vi "DO Tristate with DI.vi"() -> ()   [LabVIEW 2011]
uses:
  <vilib>/DAQmx/write.llb/DAQmx Write (Digital Bool 1Line 1Point).vi
  <vilib>/DAQmx/read.llb/DAQmx Read (Digital Bool 1Line 1Point).vi
  <vilib>/DAQmx/create/channels.llb/DAQmx Create Channel (DO-Digital Output).vi
  <vilib>/DAQmx/miscellaneous.llb/DAQmx Fill In Error Info.vi
  <vilib>/DAQmx/create/channels.llb/DAQmx Create Channel (DI-Digital Input).vi
panel:
  in  "State to Write":enum16{"Tristate", "High", "Low"}(ring)
  out "data":bool
  in  "Digital Line":tag
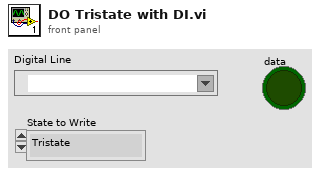
[diagram p1: front panel]
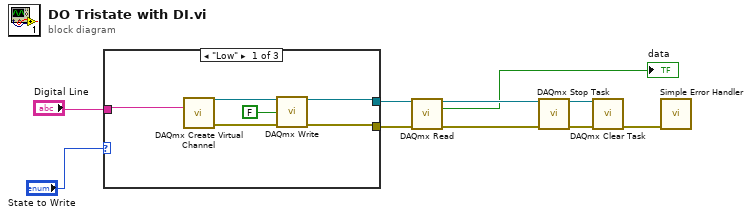
[diagram p0: block diagram]
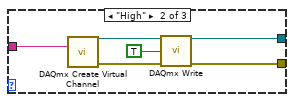
[diagram p2: hidden frame]
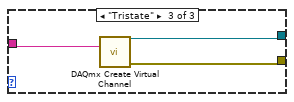
[diagram p3: hidden frame]
diagram:
  n1 = case shown="\"Low\"" "State to Write" {
    tunnel: [w12 w22 w24] -> w8
    tunnel: [w11 w21 w23] -> w7
    tunnel: "Digital Line" -> [w13 w19 w25]
    frame "Low" {
      n2 = call-poly <vilib>:"DAQmx Create Virtual Channel.vi"("lines"=w13) -> ("task out"=w14:refnum<k21>, "error out"=w15:errorcluster)  [unwired: 13 in]
      n3 = call-poly <vilib>:"DAQmx Write.vi"("task/channels in"=w14, "data"=FALSE, "error in"=w15) -> ("task out"=w12:refnum<k21>, "error out"=w11:errorcluster)  [unwired: 10 in, 1 out]
    }
    frame "High" {
      n4 = call-poly <vilib>:"DAQmx Create Virtual Channel.vi"("lines"=w19) -> ("task out"=w17:refnum<k21>, "error out"=w18:errorcluster)  [unwired: 13 in]
      n5 = call-poly <vilib>:"DAQmx Write.vi"("task/channels in"=w17, "data"=TRUE, "error in"=w18) -> ("task out"=w22:refnum<k21>, "error out"=w21:errorcluster)  [unwired: 10 in, 1 out]
    }
    frame "Tristate" {
      n6 = call-poly <vilib>:"DAQmx Create Virtual Channel.vi"("lines"=w25) -> ("task out"=w24:refnum<k21>, "error out"=w23:errorcluster)  [unwired: 13 in]
    }
  }
  n7 = call-poly <vilib>:"DAQmx Read.vi"("task/channels in"=w8, "error in"=w7) -> ("task out"=w10:refnum<k21>, "data"=→"data":bool, "error out"=w9:errorcluster)  [unwired: 11 in]
  n8 = call <vilib>:"DAQmx Stop Task.vi"("task/channels in"=w10, "error in"=w9) -> ("task out"=w5:refnum<k21>, "error out"=w4:errorcluster)  [unwired: 12 in]
  n9 = call <vilib>:"DAQmx Clear Task.vi"("task in"=w5, "error in"=w4) -> ("error out"=w3:errorcluster)  [unwired: 13 in]
  n10 = call <vilib>:"Simple Error Handler.vi"("error in (no error)"=w3) -> ()  [unwired: 4 in, 5 out]
